vi "Check Config for Active Positions.vi"(2 "Run FilePath":string, 3 "Rack Number":i8, 4 "Max Osc Per Rack":u16, 5 "AutoAge.ini  File Path":path) -> (0 "Active Positions":bool[](array[boolean]), 1 "Enabled Positions":bool[](array[boolean]))   [LabVIEW 2021]
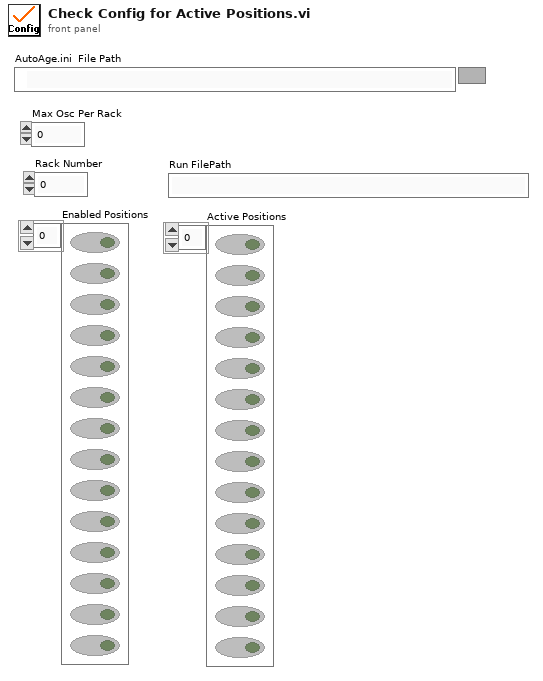
[diagram p1: front panel]
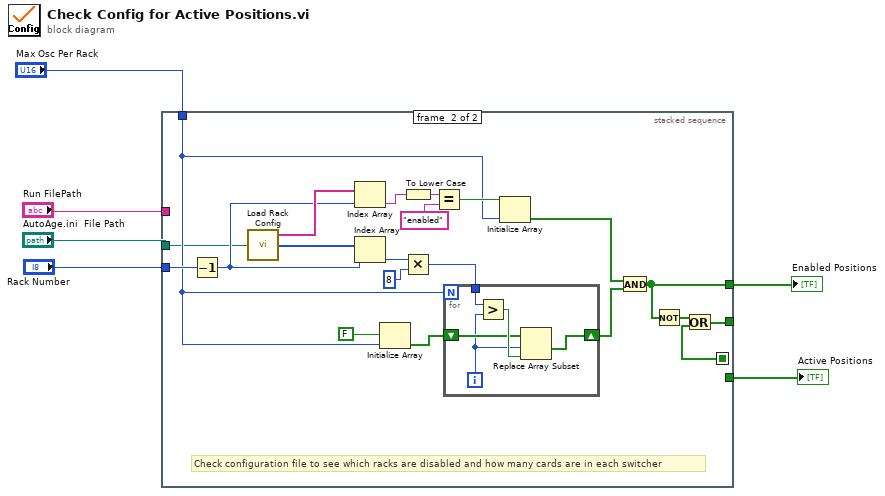
[diagram p0: block diagram]
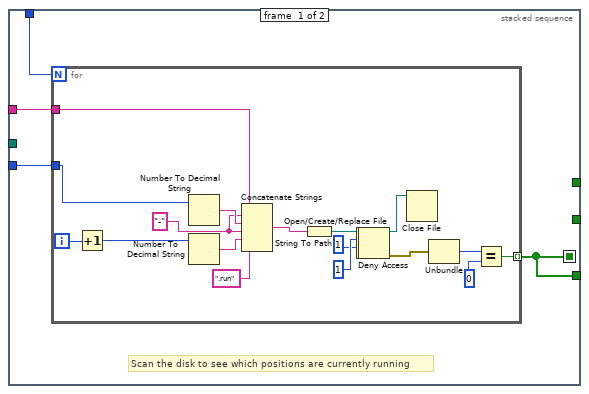
[diagram p2: hidden frame]
diagram:
  n1 = stacked-sequence {
    seq-local: [w7 _] -> [_ w36]
    tunnel: "Rack Number" -> [w10 w44]
    tunnel: [_ w35] -> _
    tunnel: "AutoAge.ini  File Path" -> [_ w33]
    tunnel: "Run FilePath" -> [w9 _]
    tunnel: "Max Osc Per Rack" -> [w8 w39]
    tunnel: [w7 _] -> w2
    tunnel: [_ w30] -> w1
    frame #0 {
      # "Scan the disk to see which positions are currently running"
      n2 = for {
        N: w8 -> [_]
        tunnel: [w28] -> w7 mode=indexing
        tunnel: w10 -> [w16]
        tunnel: w9 -> [w13]
        i -> [w29]
        w14 = "-"
        n3 = Increment(x=w29) -> (x+1=w17:i32)
        n4 = Number To Decimal String(number=w16) -> (decimal integer string=w20:string)  [unwired: 1 in]
        n5 = Number To Decimal String(number=w17) -> (decimal integer string=w19:string)  [unwired: 1 in]
        n6 = Concatenate Strings(w13, w14, w20, w14, w19, ".run") -> (w18:string)
        n7 = String To Path(string=w18) -> (path=w27:path)
        n8 = Open/Create/Replace File(file path (use dialog)=w27, access (0:read/write)=1) -> (refnum out=w11:refnum<file>, error out=w12:errorcluster)  [unwired: 4 in, 1 out]
        n9 = Deny Access(4:w12, 6:1, 7:w11) -> (0:w24:errorcluster, 3:w21:refnum<file>)
        n10 = Close File(refnum=w21) -> ()  [unwired: 1 in, 2 out]
        n11 = Unbundle(w24) -> ("code"=w22:i32)  [unwired: 2 out]
        n12 = Equal?(x=w22, y=0) -> (x = y?=w28:bool)
      }
    }
    frame #1 {
      # "Check configuration file to see which racks are disabled and how many cards are in each switcher"
      n13 = Decrement(x=w44) -> (x-1=w34:i8)
      n14 = call "Load Rack Config"("AutoAge.ini  File Path"=w33) -> ("Rack Status"=w45:string[], "# of Cards"=w49:i32[])  [unwired: 1 out]
      n15 = Index Array(array=w45, index=w34) -> (element=w43:string)
      n16 = Index Array(array=w49, index=w34) -> (element=w50:i32)
      n17 = Initialize Array(FALSE, w39) -> (w40:bool[])
      n18 = To Lower Case(string=w43) -> (all lower case string=w48:string)
      n19 = Multiply(x=w50, y=8) -> (x*y=w41:i32)
      n20 = Equal?(x=w48, y="enabled") -> (x = y?=w42:bool)
      n21 = for {
        N: w39 -> [_]
        tunnel: w41 -> [w55]
        shift-right: [w52] -> w37
        shift-left: w40 -> [w53]
        i -> [w51]
        n22 = Greater?(x=w55, y=w51) -> (0:w54:bool)
        n23 = Replace Array Subset(array=w53, new element=w54, index=w51) -> (w52:bool[])
      }
      n24 = Initialize Array(w42, w39) -> (w38:bool[])
      n25 = And(x=w38, y=w37) -> (x .and. y?=w30:bool[])
      n26 = Not(x=w30) -> (.not. x?=w31:bool[])
      n27 = Or(x=w31, y=w36) -> (x .or. y?=w35:bool[])
    }
  }
  "Active Positions" <- w2
  "Enabled Positions" <- w1
